vi "N9310A LF Out.vi"() -> ()   [LabVIEW 2018]
uses:
  <instrlib>/Agilent N9310/Agilent N9310.lvlib
panel:
  in  "Stop":bool
  in  "LF output":bool
  in  "Amplitude (V)":dbl format="%#_6p"
  in  "VISA resource name":refnum<visa-resource-name>
  in  "Frequency (Hz)":dbl format="%#_6p"
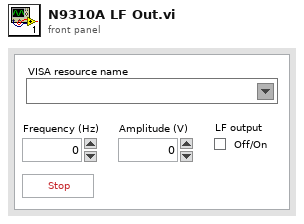
[diagram p1: front panel]
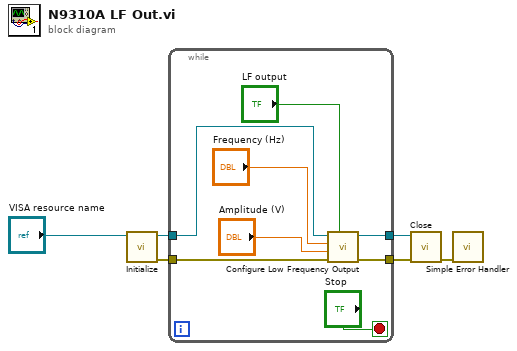
[diagram p0: block diagram]
diagram:
  n1 = call <instrlib>:"Initialize.vi"("VISA resource name"="VISA resource name") -> ("error out"=w5:errorcluster, "VISA resource name out"=w4:refnum<visa-resource-name>)  [unwired: 9 in]
  n2 = while {
    tunnel: w5 -> [w13]
    tunnel: w4 -> [w12]
    tunnel: [w9] -> w3
    tunnel: [w8] -> w2
    stop <- "Stop" stop-if-true
    n3 = call <instrlib>:"Configure Low Frequency Output.vi"("Enable LF Output (F:Disable)"="LF output", "error in (no error)"=w13, "Amplitude (0.5 V)"="Amplitude (V)", "Frequency (1.0 kHz)"="Frequency (Hz)", "VISA resource name"=w12) -> ("error out"=w9:errorcluster, "VISA resource name out"=w8:refnum<visa-resource-name>)  [unwired: 5 in]
  }
  n4 = call <instrlib>:"Close.vi"("error in (no error)"=w3, "VISA resource name"=w2) -> ("error out"=w1:errorcluster)  [unwired: 9 in]
  n5 = call <vilib>:"Simple Error Handler.vi"("error in (no error)"=w1) -> ()  [unwired: 4 in, 5 out]
